vi "Reference Queue (Array).vi"(6 "Priority Message? (F)":bool[](array[boolean]), 8 "error in (no error)":errorcluster, 9 "timeout in ms (-1)":i32=-1, 10 "Message Data":variant[](array[variant]), 11 "Tasks":T1[](array[typedef])) -> (0 "error out":errorcluster)   [LabVIEW 2019, in "Message Queue.lvlib"]
doc: "Function to enqueue a Message in a Queue of other Module."
uses:
  Message Queue.lvlib
  State Name.ctl
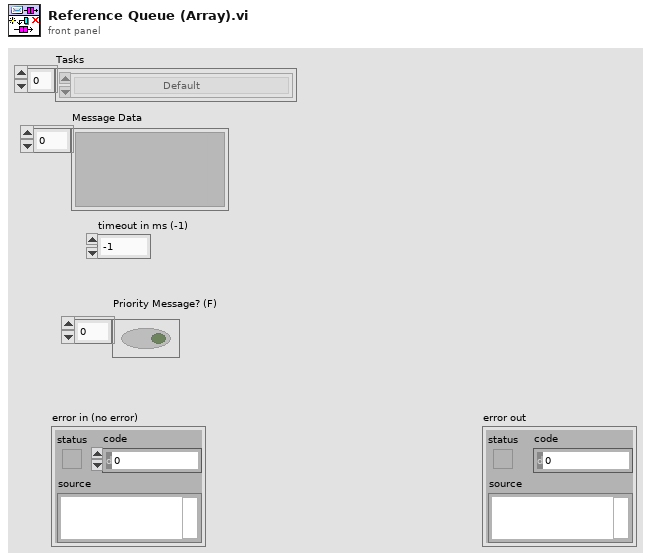
[diagram p1: front panel]
types:
  T1 = typedef "Message Queue.lvlib/State Name.ctl" = enum16{"Default", "Initialize", "Initialize Data", "Initialize Modules", "Initialize Panel", "Close FP", "Open FP", "Initialize Menu", "Mode", "Update Subpanel", "Error", "Open Help", "About", "Open WebResources", "Exit"}
  T2 = typedef "Message Queue Ref.ctl" = refnum<queue>
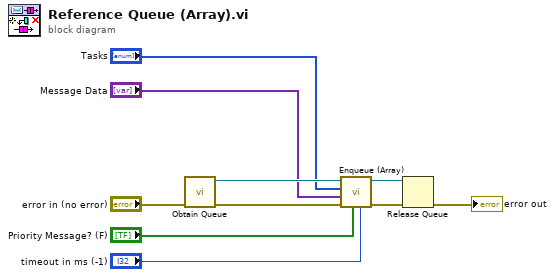
[diagram p0: block diagram]
diagram:
  n1 = call "Obtain Queue.vi"("error in (no error)"="error in (no error)") -> ("error out"=w6:errorcluster, "Message Queue out"=w8:T2)  [unwired: 9 in]
  n2 = call "Enqueue (Array).vi"("timeout in ms (-1)"="timeout in ms (-1)", "Priority Message? Array"="Priority Message? (F)", "error in (no error)"=w6, "Message Data Array"="Message Data", "States"="Tasks", "Message Queue"=w8) -> ("error out"=w1:errorcluster, "dup Message Queue"=w2:T2)  [unwired: 4 in]
  n3 = Release Queue(queue=w2, error in (no error)=w1) -> (error out=→"error out":errorcluster)  [unwired: 1 in, 2 out]
